vi "SCM1 Control.vi"() -> ()   [LabVIEW 2021]
doc: "Modified from Hannahs' General GPIB Transaction to deal with Oxford's use of carrage returns rather than EOI"
panel:
  out "?":string="  "
  out "message":string="Switch heater fault!   \n(Probably disconnected)"
  out "Persistent Field \n(from PS memory)":dbl format="%.3f"
  in  "To Zero":bool
  in  "Switch Heater":bool
  in  "Ramp":bool
  out "Present Field":dbl format="%.3f"
  in  "GPIB Address":refnum<visa-resource-name>="GPIB0:25:INSTR"
  in  "Set Point":dbl min=-20.0 max=20.0 format="%.3f"
  in  "Ramp Rate":dbl=0.5 min=0.0 max=3.5 format="%.2f"
  # "Tesla"
  # "Amp/m"
  # "Ramps from present field to the Set Point (< 20 T), at the given Ramp Rate (< 3.5 A/m)."
  # "Tesla"
  # "Hold"
  # "Off"
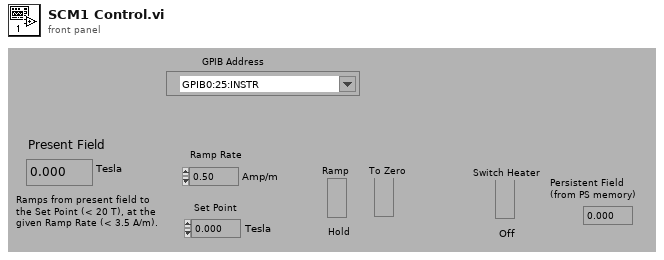
[diagram p1: front panel]
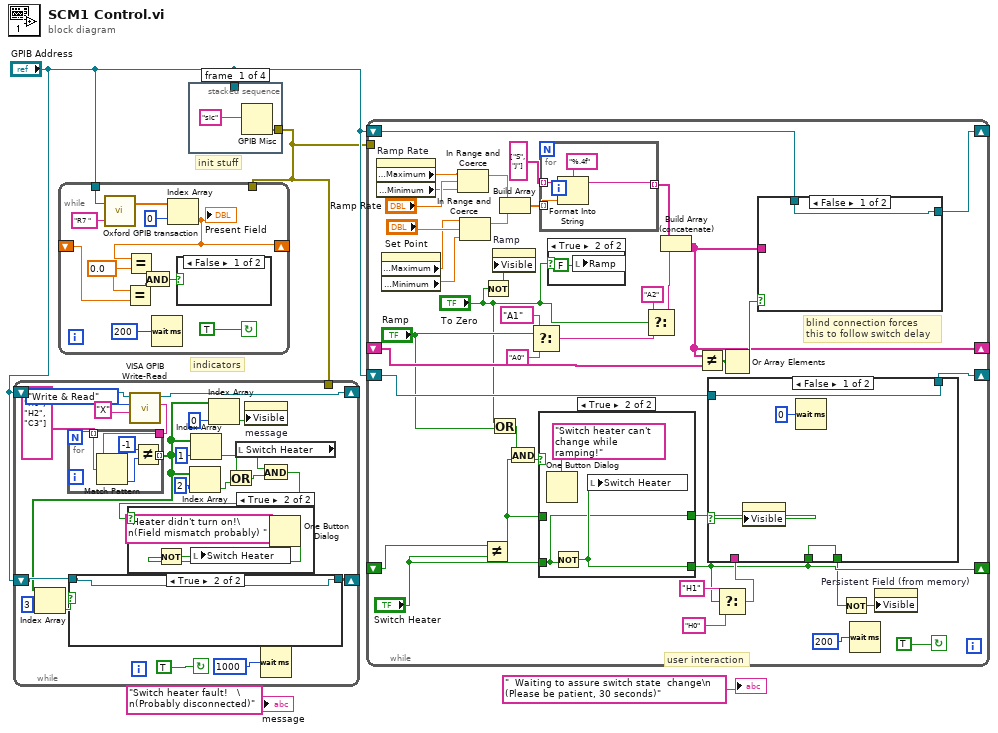
[diagram p0: block diagram]
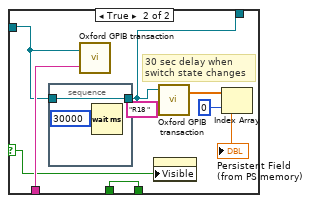
[diagram p4: hidden frame]
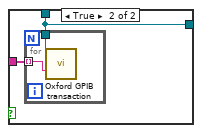
[diagram p5: hidden frame]
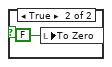
[diagram p6: hidden frame]
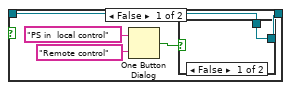
[diagram p7: hidden frame]
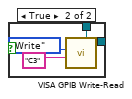
[diagram p8: hidden frame]
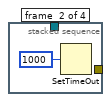
[diagram p10: hidden frame]
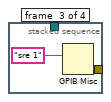
[diagram p11: hidden frame]
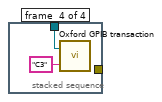
[diagram p12: hidden frame]
diagram:
  # "user interaction"
  # "indicators"
  # "init stuff"
  n1 = stacked-sequence {
    tunnel: "GPIB Address" -> [_ _ _ w10]
    tunnel: [w5 _ _ _] -> w1
    frame #0 {
      n2 = GPIB Misc(0:"sic" ("command string")) -> (4:w5:errorcluster)  [unwired: 1 in, 2 out]
    }
    frame #1 {
      n3 = SetTimeOut(1:1000 ("new timeout (10000)")) -> ()  [unwired: 1 out]
    }
    frame #2 {
      n4 = GPIB Misc(0:"sre 1") -> ()  [unwired: 1 in, 3 out]
    }
    frame #3 {
      n5 = call "Oxford GPIB transaction.vi"("Command String"="C3", "GPIB Address"=w10) -> ()  [unwired: 2 out]
    }
  }
  n6 = while {
    tunnel: w1 -> [_]
    shift-right: [w12] -> _
    shift-left: "GPIB Address" -> [w13]
    shift-right: [w11] -> _
    shift-left: "GPIB Address" -> [w27]
    stop <- TRUE continue-if-true
    n7 = call "VISA GPIB Write-Read.vi"("Command"="X", "Action"=enum16{"Write", "Read", "Write & Read"}."Write & Read", "VISA resource name"=w13) -> ("String Returned"=w14:string, "dup VISA Session"=w12:refnum<visa-resource-name>)  [unwired: 5 in, 2 out]
    n8 = for {
      tunnel: string[] ["H5", "H0", "H2", "C3"] -> [w48] mode=indexing
      tunnel: [w45] -> w19 mode=indexing
      tunnel: w14 -> [w44]
      n9 = Match Pattern(string=w44, regular expression=w48) -> (offset past match=w46:i32)  [unwired: 1 in, 3 out]
      n10 = Not Equal?(x=-1, y=w46) -> (x != y?=w45:bool)
    }
    n11 = Index Array(array=w19, index=3) -> (element=w17:bool)
    n12 = case shown="True" w17 {
      tunnel: w27 -> [w35 w43]
      tunnel: [w33 w43] -> w11
      frame False {
        n13 = One Button Dialog(message="PS in  local control", button name ("OK")="Remote control") -> (true=w34:bool)
        n14 = case shown="False" w34 {
          tunnel: w35 -> [w38 w40]
          tunnel: [w38 w39] -> w33
          frame False {
          }
          frame True {
            n15 = call "VISA GPIB Write-Read.vi"("Command"="C3" ("String to Write"), "Action"=enum16{"Write", "Read", "Write & Read"}."Write", "VISA resource name"=w40) -> ("dup VISA Session"=w39:refnum<visa-resource-name>)  [unwired: 5 in, 3 out]
          }
        }
      }
      frame True {
      }
    }
    n16 = Index Array(array=w19, index=2) -> (element=w21:bool)
    n17 = Index Array(array=w19, index=1) -> (element=w22:bool)
    n18 = Index Array(array=w19, index=0) -> (element=w26:bool)
    n19 = Or(x=w22, y=w21) -> (x .or. y?=w30:bool)
    n20 = local read "Switch Heater"() -> (w29:bool)
    n21 = property on="message" class="Str"("Visible"=w26) -> ()  [unwired: 2 in, 2 out]
    n22 = And(x=w29, y=w30) -> (x .and. y?=w18:bool)
    n23 = case shown="True" w18 {
      frame False {
      }
      frame True {
        n24 = One Button Dialog(message="Heater didn't turn on!\n(Field mismatch probably) ") -> (true=w49:bool)  [unwired: 1 in]
        n25 = Not(x=w49) -> (.not. x?=w50:bool)
        n26 = local write "Switch Heater"(w50) -> ()
      }
    }
    n27 = Wait (ms)(milliseconds to wait=1000) -> ()  [unwired: 1 out]
  }
  n28 = while {
    shift-left: _ -> [w52]
    shift-right: [w56] -> _
    tunnel: w1 -> [_]
    tunnel: "GPIB Address" -> [w61]
    stop <- TRUE continue-if-true
    w57 = 0.0 ("y")
    n29 = call "Oxford GPIB transaction.vi"("Command String"="R7 ", "GPIB Address"=w61) -> ("Measurement"=w59:dbl[])  [unwired: 1 out]
    n30 = Equal?(x=w57, y=w52) -> (x = y?=w54:bool)
    n31 = Wait (ms)(milliseconds to wait=200) -> ()  [unwired: 1 out]
    n32 = Index Array(array=w59, index=0) -> (element=w56:dbl)
    "Present Field" <- w56
    n33 = Equal?(x=w56, y=w57) -> (x = y?=w55:bool)
    n34 = And(x=w55, y=w54) -> (x .and. y?=w53:bool)
    n35 = case shown="False" w53 {
      frame False {
      }
      frame True {
        n36 = local write "To Zero"(FALSE ("To Zero")) -> ()
      }
    }
  }
  n37 = while {
    shift-left: _ -> [w81]
    shift-right: [w76] -> _
    tunnel: w1 -> [_]
    shift-left: _ -> [w92]
    shift-right: [w93] -> _
    shift-right: [w66] -> _
    shift-left: "GPIB Address" -> [w91]
    shift-right: [w65] -> _
    shift-left: "GPIB Address" -> [w94]
    stop <- TRUE continue-if-true
    # "blind connection forces \nthis to follow switch delay"
    n38 = property on="Ramp Rate" class="DigNum (strict)"() -> ("Data Range:Maximum"=w71:dbl, "Data Range:Minimum"=w70:dbl)  [unwired: 2 in, 2 out]
    n39 = property on="Set Point" class="DigNum (strict)"() -> ("Data Range:Maximum"=w68:dbl, "Data Range:Minimum"=w67:dbl)  [unwired: 2 in, 2 out]
    n40 = In Range and Coerce(upper limit=w71, x="Ramp Rate", lower limit=w70) -> (coerced(x)=w74:dbl)  [unwired: 1 out]
    n41 = In Range and Coerce(upper limit=w68, x="Set Point", lower limit=w67) -> (coerced(x)=w72:dbl)  [unwired: 1 out]
    n42 = Not Equal?(x=w81, y="Switch Heater") -> (x != y?=w79:bool)
    n43 = Not(x="To Zero") -> (.not. x?=w86:bool)
    n44 = Or(x="To Zero", y="Ramp") -> (x .or. y?=w83:bool)
    n45 = property on="Ramp" class="Bool (strict)"("Visible"=w86) -> ()  [unwired: 2 in, 2 out]
    n46 = Build Array(w74, w72) -> (w101:dbl[])
    n47 = And(x=w83, y=w79) -> (x .and. y?=w82:bool)
    n48 = Select(t="A1", s="Ramp", f="A0") -> (s? t:f=w89:string)
    n49 = case shown="True" w82 {
      tunnel: [w107 w108] -> w80
      tunnel: w79 -> [w107 _]
      tunnel: "Switch Heater" -> [w106 w108]
      tunnel: [w106 w109] -> w76
      frame False {
      }
      frame True {
        n50 = One Button Dialog(message="Switch heater can't change while ramping!") -> ()  [unwired: 1 in, 1 out]
        n51 = Not(x=w108) -> (.not. x?=w109:bool)
        n52 = local write "Switch Heater"(w109) -> ()
      }
    }
    n53 = for {
      tunnel: w101 -> [w134] mode=indexing
      tunnel: string[] ["S", "J"] -> [w133] mode=indexing
      tunnel: [w132] -> w104 mode=indexing
      n54 = Format Into String(format string="%.4f", initial string=w133, w134) -> (resulting string=w132:string)  [unwired: 1 in, 1 out]
    }
    n55 = case shown="True" "To Zero" {
      frame False {
      }
      frame True {
        n56 = local write "Ramp"(FALSE ("Ramp")) -> ()
      }
    }
    n57 = Select(t="A2", s="To Zero", f=w89) -> (s? t:f=w90:string)
    n58 = Build Array (concatenate)(w104, w90) -> (w93:string[])
    n59 = Not Equal?(x=w93, y=w92) -> (x != y?=w98:bool[])
    n60 = Select(t="H1", s=w76, f="H0") -> (s? t:f=w78:string)
    n61 = case shown="False" w80 {
      selector: w80 -> [w114 w117]
      tunnel: w91 -> [w112 w119]
      tunnel: w78 -> [_ w124]
      tunnel: [w112 w118] -> w66
      tunnel: w76 -> [w113 w116]
      tunnel: [w113 w116] -> w75
      frame False {
        n62 = property class="Str"("Visible"=w114) -> ()  [unwired: 2 in, 2 out]
        n63 = Wait (ms)(milliseconds to wait=u32 0) -> ()  [unwired: 1 out]
      }
      frame True {
        # "30 sec delay when \nswitch state changes"
        n64 = stacked-sequence {
          tunnel: [w125] -> w118
          tunnel: w119 -> [w125]
          frame #0 {
            n65 = Wait (ms)(milliseconds to wait=u32 30000) -> ()  [unwired: 1 out]
          }
        }
        n66 = call "Oxford GPIB transaction.vi"("Command String"=w124, "GPIB Address"=w119) -> ()  [unwired: 2 out]
        n67 = property class="Str"("Visible"=w117) -> ()  [unwired: 2 in, 2 out]
        n68 = call "Oxford GPIB transaction.vi"("Command String"="R18 ", "GPIB Address"=w118) -> ("Measurement"=w122:dbl[])  [unwired: 1 out]
        n69 = Index Array(array=w122, index=0) -> (element=→"Persistent Field \n(from PS memory)":dbl)
      }
    }
    n70 = Or Array Elements(Boolean array=w98) -> (logical OR=w95:bool)
    n71 = case shown="False" w95 {
      tunnel: w94 -> [w127 w128]
      tunnel: w93 -> [_ w129]
      tunnel: [w127 w128] -> w65
      frame False {
      }
      frame True {
        n72 = for {
          tunnel: w128 -> [w131]
          tunnel: w129 -> [w130] mode=indexing
          n73 = call "Oxford GPIB transaction.vi"("Command String"=w130, "GPIB Address"=w131) -> ()  [unwired: 2 out]
        }
      }
    }
    n74 = Not(x=w75) -> (.not. x?=w87:bool)
    n75 = Wait (ms)(milliseconds to wait=200) -> ()  [unwired: 1 out]
    n76 = property on="Persistent Field (from memory)" class="DigNum (strict)"("Visible"=w87) -> ()  [unwired: 2 in, 2 out]
  }
  "message" <- "Switch heater fault!   \n(Probably disconnected)" ("message")
  "?" <- "  Waiting to assure switch state  change\n        (Please be patient, 30 seconds)"
